vi "Scripting_CheckIfErrorCluster.vi"(8 "error in (no error)":errorcluster, 11 "Ctl Refnum":refnum<vi>) -> (0 "error out":errorcluster, 2 "IsErrClust?":bool, 3 "Ctl Refnum 2":refnum<vi>)   [LabVIEW 2012]
uses:
  <vilib>/Utility/VariantDataType/Type.ctl
  <vilib>/Utility/VariantDataType/VariantType.lvlib
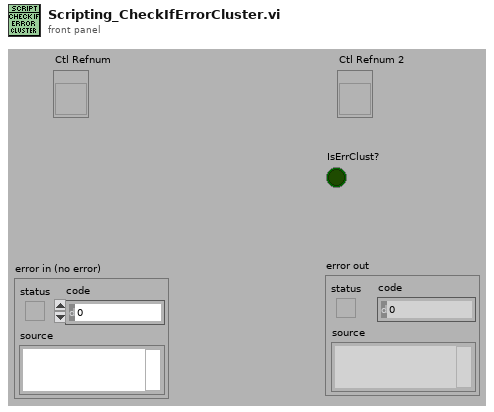
[diagram p1: front panel]
types:
  T1 = typedef "VariantType.lvlib/Type.ctl" = enum8{"Invalid Type", "Void", "I8", "I16", "I32", "I64", "U8", "U16", "U32", "U64", "Single Float", "Double Float", "Extended Float", "Single Complex", "Double Complex", "Extended Complex", "Enum U8", "Enum U16", "Enum U32", "Enum U64", "Single Float With Unit", "Double Float With Unit", "Extended Float With Unit", "Single Complex with Unit", "Double Complex with Unit", "Extended Complex with Unit", "Boolean", "String", "Path", "Picture", "Tag", "Array", "Cluster", "Variant", "LV Variant", "Waveform", "Timestamp", "Digital Waveform", "Digital Data", "ExpressData", "Refnum", "External Data", "VI", "Poly VI", "LabVIEW Class Instance", "Fixed Point"}
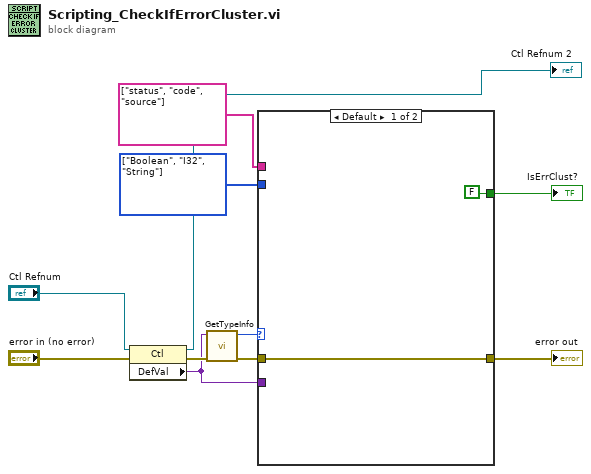
[diagram p0: block diagram]
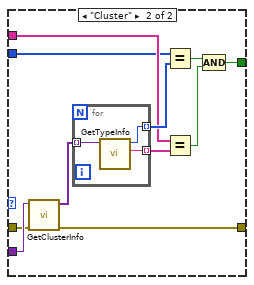
[diagram p2: hidden frame]
diagram:
  w5 = T1[] [enum."Boolean", enum."I32", enum."String"] items=["Invalid Type", "Void", "I8", "I16", "I32", "I64", "U8", "U16", "U32", "U64", "Single Float", "Double Float", "Extended Float", "Single Complex", "Double Complex", "Extended Complex", "Enum U8", "Enum U16", "Enum U32", "Enum U64", "Single Float With Unit", "Double Float With Unit", "Extended Float With Unit", "Single Complex with Unit", "Double Complex with Unit", "Extended Complex with Unit", "Boolean", "String", "Path", "Picture", "Tag", "Array", "Cluster", "Variant", "LV Variant", "Waveform", "Timestamp", "Digital Waveform", "Digital Data", "ExpressData", "Refnum", "External Data", "VI", "Poly VI", "LabVIEW Class Instance", "Fixed Point"]
  n1 = property class="Ctl"(reference="Ctl Refnum", error in="error in (no error)") -> (reference out=→"Ctl Refnum 2":refnum<vi>, error out=w10:errorcluster, "DefVal"=w8:variant)
  n2 = call <vilib>:"GetTypeInfo.vi"("error in (no error)"=w10, "Variant"=w8) -> ("error out"=w9:errorcluster, "Type Enum"=w11:T1)  [unwired: 5 in, 3 out]
  n3 = case shown="Default" w11 {
    tunnel: w8 -> [_ w24]
    tunnel: string[] ["status", "code", "source"] -> [_ w20]
    tunnel: w5 -> [_ w19]
    tunnel: [FALSE w16] -> w1
    tunnel: w9 -> [w13 w15]
    tunnel: [w13 w14] -> w3
    frame Default {
    }
    frame "Cluster" {
      n4 = call <vilib>:"GetClusterInfo.vi"("error in (no error)"=w15, "Variant"=w24) -> ("error out"=w14:errorcluster, "Cluster Elements"=w23:variant[])  [unwired: 8 in]
      n5 = for {
        tunnel: w23 -> [w27] mode=indexing
        tunnel: [w26] -> w22 mode=indexing
        tunnel: [w25] -> w21 mode=indexing
        n6 = call <vilib>:"GetTypeInfo.vi"("Variant"=w27) -> ("Name"=w25:string, "Type Enum"=w26:T1)  [unwired: 6 in, 3 out]
      }
      n7 = Equal?(x=w19, y=w22) -> (x = y?=w18:bool)
      n8 = Equal?(x=w20, y=w21) -> (x = y?=w17:bool)
      n9 = Compound Arithmetic op=AND(w18, w17) -> (w16:bool)
    }
  }
  "error out" <- w3
  "IsErrClust?" <- w1
